vi "cmc-coin_flipper.vi"() -> ()   [LabVIEW 2010]
panel:
  out "Elapsed Time (sec)":dbl
  out "Number of Flips":u32
  in  "stop":bool
  out "Tails":u64(slide) scale=0.0..33.0
  out "Heads":u64(slide) scale=0.0..33.0
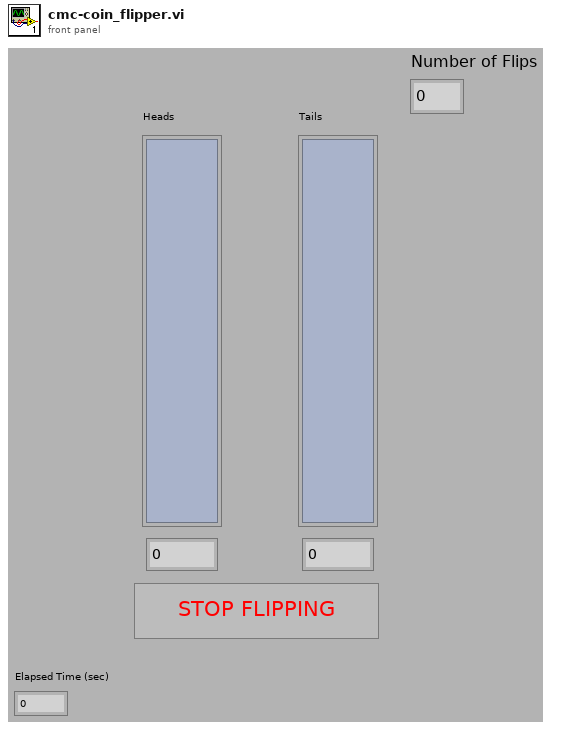
[diagram p1: front panel]
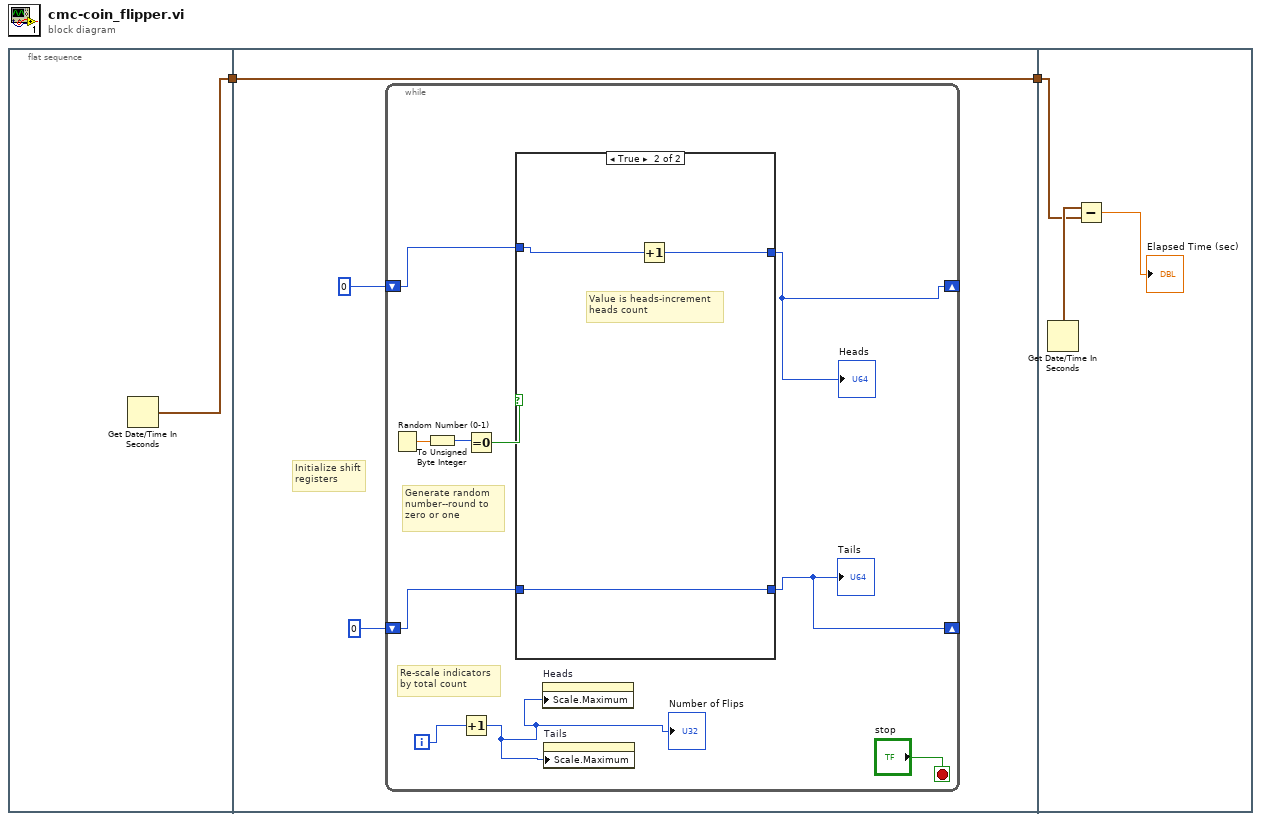
[diagram p0: block diagram]
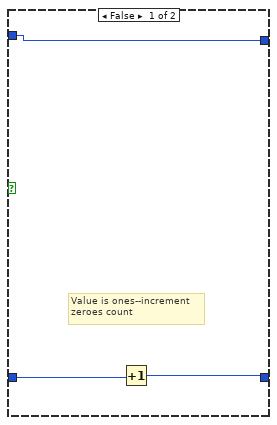
[diagram p2: hidden frame]
diagram:
  n1 = flat-sequence {
    tunnel: [w3] -> w2
    tunnel: w2 -> [w4]
    tunnel: [w4] -> w1
    tunnel: w1 -> [w23]
    frame #0 {
      n2 = Get Date/Time In Seconds() -> (seconds since 1Jan1904=w3:timestamp)
    }
    frame #1 {
      # "Initialize shift\nregisters"
      n3 = while {
        shift-right: [w10] -> _
        shift-left: 0 -> [w16]
        shift-right: [w9] -> _
        shift-left: 0 -> [w15]
        i -> [w8]
        stop <- "stop" stop-if-true
        # "Re-scale indicators\nby total count"
        # "Generate random\nnumber--round to\nzero or one"
        n4 = Random Number (0-1)() -> (number: 0 to 1=w14:dbl)
        n5 = To Unsigned Byte Integer(number=w14) -> (unsigned 8bit integer=w13:u8)
        n6 = Increment(x=w8) -> (x+1=w7:i32)
        "Number of Flips" <- w7
        n7 = Equal To 0?(x=w13) -> (x = 0?=w12:bool)
        n8 = case shown="True" w12 {
          tunnel: w16 -> [w19 w22]
          tunnel: w15 -> [w18 w20]
          tunnel: [w19 w21] -> w10
          tunnel: [w17 w20] -> w9
          frame False {
            # "Value is ones--increment\nzeroes count"
            n9 = Increment(x=w18) -> (x+1=w17:i32)
          }
          frame True {
            # "Value is heads-increment\nheads count"
            n10 = Increment(x=w22) -> (x+1=w21:i32)
          }
        }
        "Tails" <- w9
        "Heads" <- w10
        n11 = property on="Heads" class="Slide (strict)"("Scale.Maximum"=w7) -> ()  [unwired: 2 in, 2 out]
        n12 = property on="Tails" class="Slide (strict)"("Scale.Maximum"=w7) -> ()  [unwired: 2 in, 2 out]
      }
    }
    frame #2 {
      n13 = Get Date/Time In Seconds() -> (seconds since 1Jan1904=w24:timestamp)
      n14 = Subtract(x=w24, y=w23) -> (x-y=→"Elapsed Time (sec)":dbl)
    }
  }
